vi "main.vi"() -> ()   [LabVIEW 2023]
uses:
  TypeDefs/States.ctl
  subVIs/Open_device.llb/Select_Instr.ctl
  <vilib>/Analysis/1siggen.llb/Ramp Pattern by Samples.vi
  <vilib>/Analysis/NI_AALBase.lvlib
panel:
  in  "f_start [Hz]":dbl=1.0 min=1.0 max=1000.0 format="%0.2f"
  in  "f_stop [Hz]":dbl=1.0 min=1.0 max=10000.0
  in  "samples":i32=128 min=1 max=1000
  out "Jeden punkt pomiarowy":cluster{dbl, dbl}
  out "Modul i faza impedancji":cluster{dbl, dbl}[](graph)
  out "Cosinus fi":dbl
  out "Uwagi do pomiarów":string
  out "|Z|":dbl
  out "U3 [V]":dbl format="%#.3g"
  out "U2 [V]":dbl format="%#.3g"
  out "U1 [V]":dbl format="%#.3g"
  in  "Pomiar":bool
  in  "stop":bool
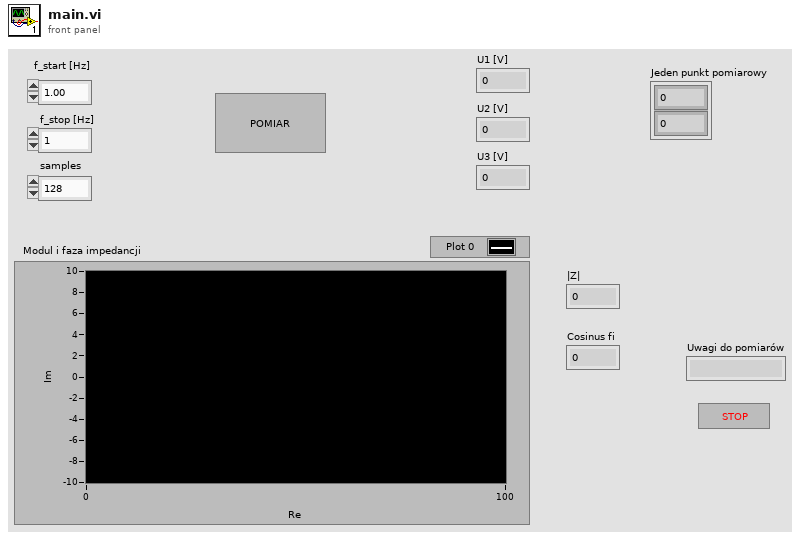
[diagram p1: front panel]
types:
  T1 = typedef "States.ctl" = enum16{"INIT", "WAIT", "EXIT", "GEN", "MEAS1", "MEAS2", "MEAS3", "CALC"}
  T2 = typedef "Select_Instr.ctl" = string
  T3 = cluster{"VISA resource name 1":refnum<visa-resource-name>, "VISA resource name 2":refnum<visa-resource-name>, "VISA resource name 3":refnum<visa-resource-name>}
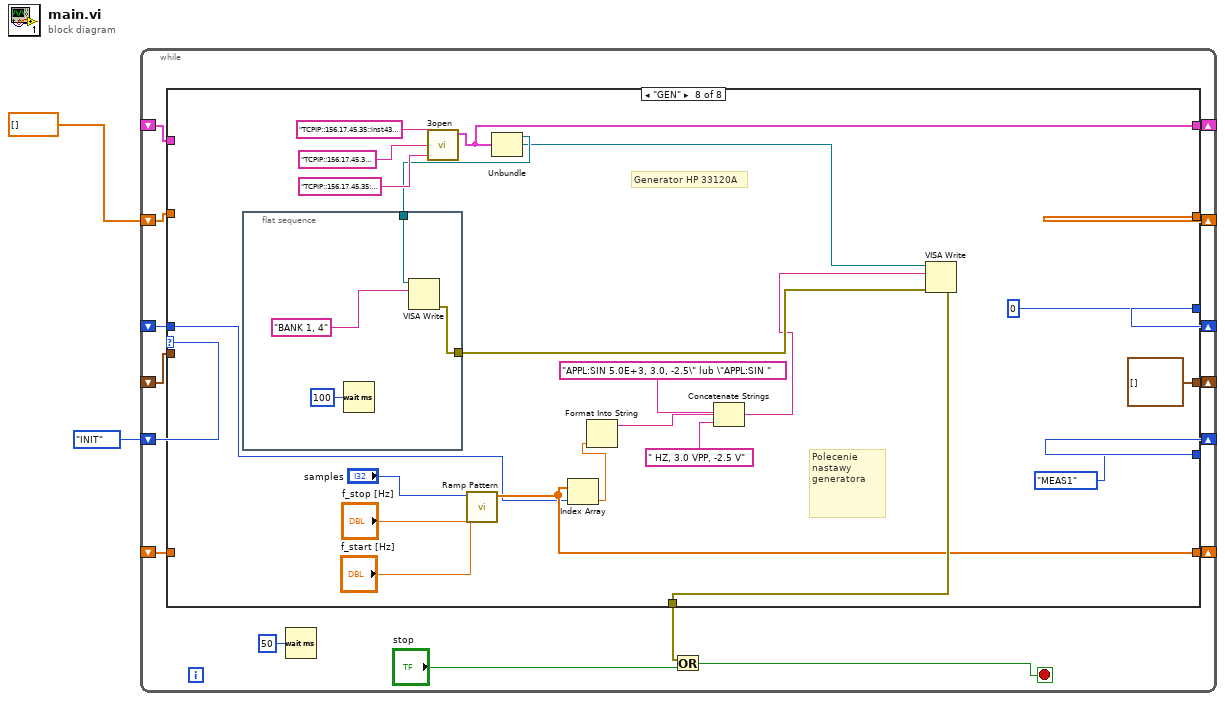
[diagram p0: block diagram]
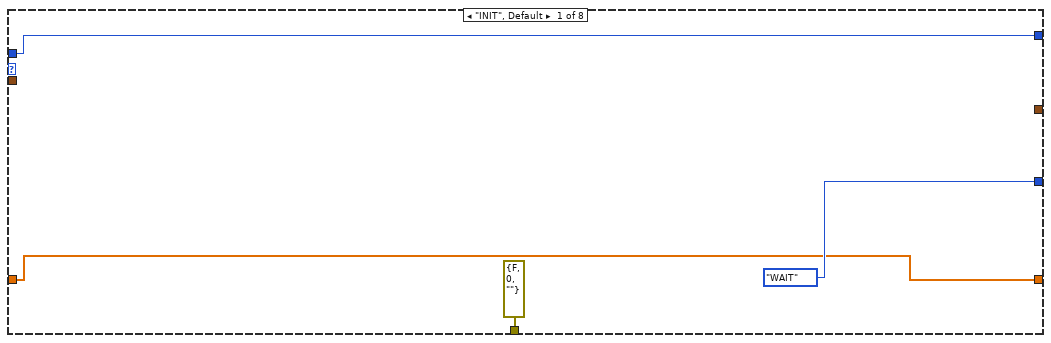
[diagram p2: hidden frame]
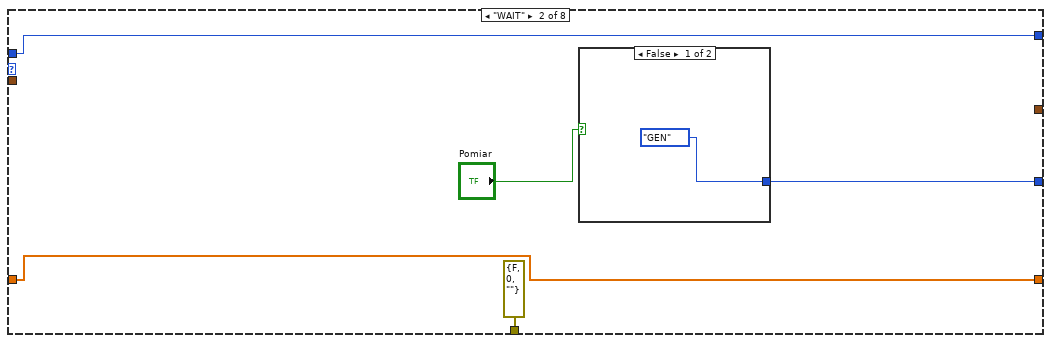
[diagram p3: hidden frame]
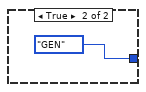
[diagram p4: hidden frame]
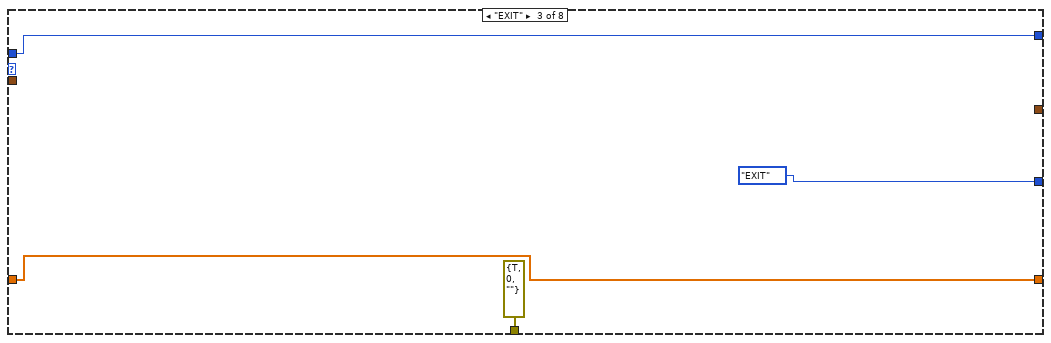
[diagram p5: hidden frame]
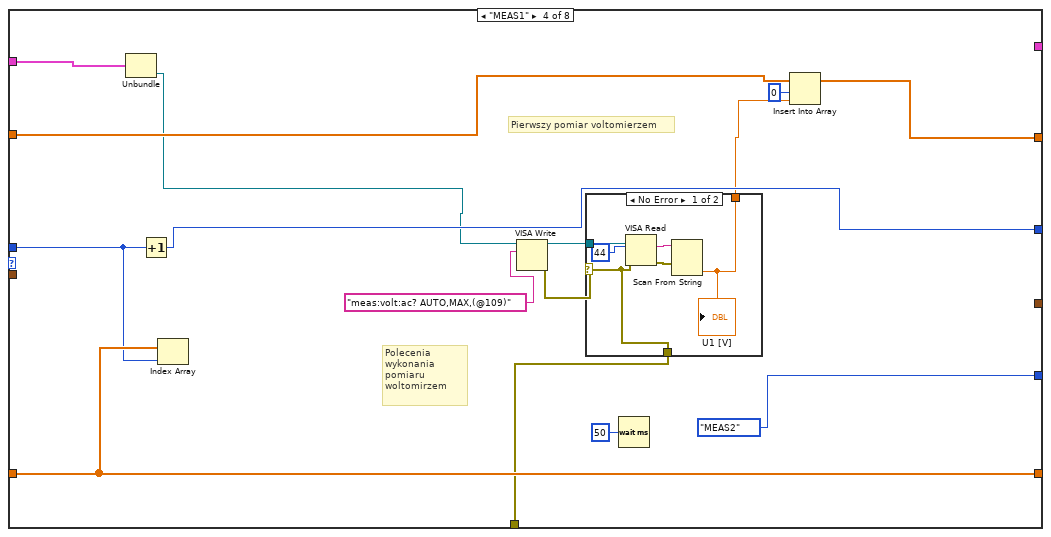
[diagram p6: hidden frame]
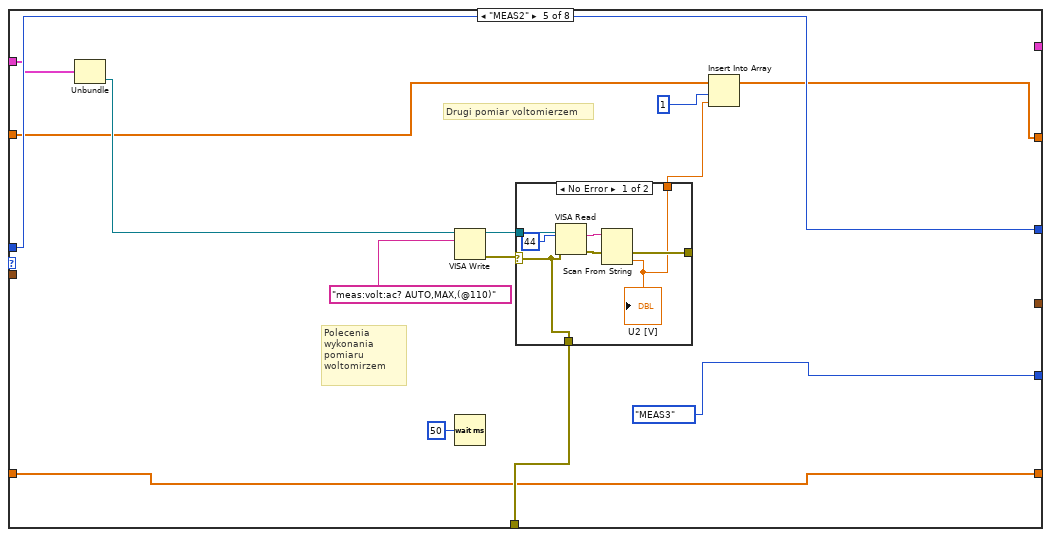
[diagram p8: hidden frame]
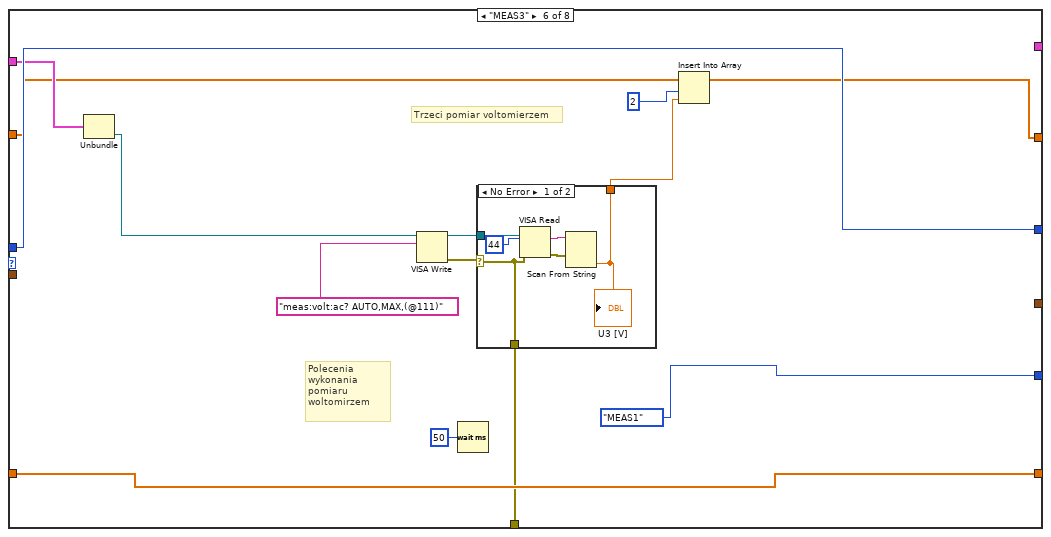
[diagram p10: hidden frame]
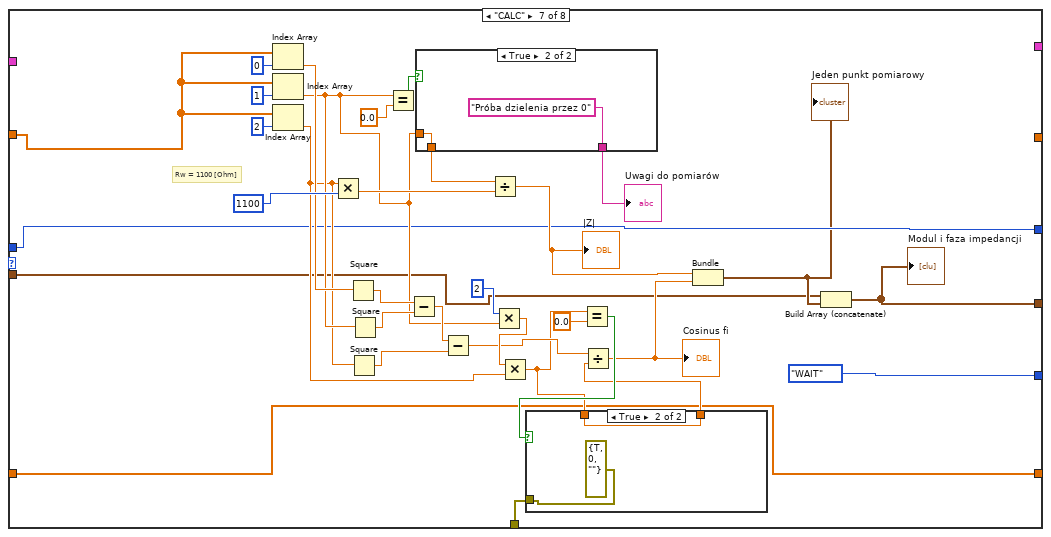
[diagram p12: hidden frame]
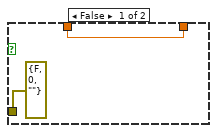
[diagram p13: hidden frame]
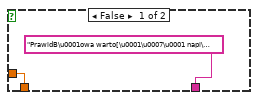
[diagram p14: hidden frame]
diagram:
  n1 = while {
    shift-right: [w18] -> _
    shift-left: States."INIT" -> [w17]
    shift-right: [w13] -> _
    shift-left: dbl[] [] -> [w12]
    shift-right: [w10] -> _
    shift-left: _ -> [w9]
    shift-right: [w8] -> _
    shift-left: _ -> [w6]
    shift-right: [w7] -> _
    shift-left: _ -> [w5]
    shift-right: [w4] -> _
    shift-left: _ -> [w3]
    stop <- w14 stop-if-true
    n2 = case shown="\"GEN\"" w17 {
      tunnel: [States."WAIT" w26 States."EXIT" States."MEAS2" States."MEAS3" States."MEAS1" States."WAIT" States."MEAS1"] -> w18
      tunnel: [errorcluster {"status"=FALSE, "code"=0, "source"=""} ("error IO") errorcluster {"status"=FALSE, "code"=0, "source"=""} ("error IO") errorcluster {"status"=TRUE, "code"=0, "source"=""} ("error IO") w35 w68 w82 w109 w148] -> w16
      tunnel: [_ _ _ w36 w56 w78 _ _] -> w13
      tunnel: w12 -> [_ _ _ w39 w59 w79 w102 _]
      tunnel: [_ _ _ _ _ _ _ w153] -> w10
      tunnel: w9 -> [_ _ _ w47 w61 w84 _ _]
      tunnel: [w20 w24 w31 w46 w67 w90 w104 w146] -> w8
      tunnel: [w19 w23 w30 w40 w66 w89 w103 0] -> w7
      tunnel: w6 -> [w20 w24 w31 w46 w67 w90 w104 _]
      tunnel: w5 -> [w19 w23 w30 w45 w66 w89 w103 w140]
      tunnel: [_ _ _ _ _ _ w99 cluster{dbl, dbl}[] []] -> w4
      tunnel: w3 -> [_ _ _ _ _ _ w100 _]
      frame "INIT", Default {
      }
      frame "WAIT" {
        n3 = case shown="False" "Pomiar" {
          tunnel: [States."GEN" States."GEN"] -> w26
          frame False {
          }
          frame True {
          }
        }
      }
      frame "EXIT" {
      }
      frame "MEAS1" {
        # "Polecenia wykonania \npomiaru woltomirzem"
        # "Pierwszy pomiar voltomierzem"
        n4 = Unbundle(w47) -> ("VISA resource name 3"=w34:refnum<visa-resource-name>)  [unwired: 2 out]
        n5 = Increment(x=w45) -> (x+1=w40:i32)
        n6 = Index Array(array=w46, index=w45) -> ()  [unwired: 1 out]
        n7 = VISA Write(VISA resource name=w34, write buffer="meas:volt:ac? AUTO,MAX,(@109)") -> (VISA resource name out=w43:refnum<visa-resource-name>, error out=w42:errorcluster)  [unwired: 1 in, 1 out]
        n8 = case shown="No Error" w42 {
          selector: w42 -> [w49 w55]
          tunnel: w43 -> [w54 _]
          tunnel: [w50 _] -> w38
          tunnel: [w49 w55] -> w35
          frame No Error {
            n9 = VISA Read(VISA resource name=w54, byte count=u32 44, error in (no error)=w49) -> (read buffer=w52:string, error out=w51:errorcluster)  [unwired: 2 out]
            n10 = Scan From String(input string=w52, error in=w51) -> (output 1=w50:dbl)  [unwired: 3 in, 3 out]
            "U1 [V]" <- w50
          }
          frame Error {
          }
        }
        n11 = Wait (ms)(milliseconds to wait=u32 50) -> ()  [unwired: 1 out]
        n12 = Insert Into Array(array=w39, index=0, new element=w38) -> (w36:dbl[])
      }
      frame "MEAS2" {
        # "Polecenia wykonania \npomiaru woltomirzem"
        # "Drugi pomiar voltomierzem"
        n13 = Unbundle(w61) -> ("VISA resource name 3"=w60:refnum<visa-resource-name>)  [unwired: 2 out]
        n14 = VISA Write(VISA resource name=w60, write buffer="meas:volt:ac? AUTO,MAX,(@110)") -> (VISA resource name out=w64:refnum<visa-resource-name>, error out=w63:errorcluster)  [unwired: 1 in, 1 out]
        n15 = Wait (ms)(milliseconds to wait=u32 50) -> ()  [unwired: 1 out]
        n16 = case shown="No Error" w63 {
          selector: w63 -> [w70 w77]
          tunnel: w64 -> [w76 _]
          tunnel: [w72 w77] -> _
          tunnel: [w71 _] -> w57
          tunnel: [w70 w77] -> w68
          frame No Error {
            n17 = VISA Read(VISA resource name=w76, byte count=u32 44, error in (no error)=w70) -> (read buffer=w74:string, error out=w73:errorcluster)  [unwired: 2 out]
            n18 = Scan From String(input string=w74, error in=w73) -> (error out=w72:errorcluster, output 1=w71:dbl)  [unwired: 3 in, 2 out]
            "U2 [V]" <- w71
          }
          frame Error {
          }
        }
        n19 = Insert Into Array(array=w59, index=1, new element=w57) -> (w56:dbl[])
      }
      frame "MEAS3" {
        # "Polecenia wykonania \npomiaru woltomirzem"
        # "Trzeci pomiar voltomierzem"
        n20 = Unbundle(w84) -> ("VISA resource name 3"=w83:refnum<visa-resource-name>)  [unwired: 2 out]
        n21 = VISA Write(VISA resource name=w83, write buffer="meas:volt:ac? AUTO,MAX,(@111)") -> (VISA resource name out=w87:refnum<visa-resource-name>, error out=w86:errorcluster)  [unwired: 1 in, 1 out]
        n22 = Wait (ms)(milliseconds to wait=u32 50) -> ()  [unwired: 1 out]
        n23 = case shown="No Error" w86 {
          selector: w86 -> [w92 w98]
          tunnel: w87 -> [w97 _]
          tunnel: [w93 _] -> w80
          tunnel: [w92 w98] -> w82
          frame No Error {
            n24 = VISA Read(VISA resource name=w97, byte count=u32 44, error in (no error)=w92) -> (read buffer=w95:string, error out=w94:errorcluster)  [unwired: 2 out]
            n25 = Scan From String(input string=w95, error in=w94) -> (output 1=w93:dbl)  [unwired: 3 in, 3 out]
            "U3 [V]" <- w93
          }
          frame Error {
          }
        }
        n26 = Insert Into Array(array=w79, index=2, new element=w80) -> (w78:dbl[])
      }
      frame "CALC" {
        # "Rw = 1100 [Ohm]"
        n27 = Index Array(array=w102, index=0) -> (element=w123:dbl)
        n28 = Index Array(array=w102, index=1) -> (element=w116:dbl)
        n29 = Index Array(array=w102, index=2) -> (element=w115:dbl)
        n30 = Multiply(x=w115, y=1100) -> (x*y=w124:dbl)
        n31 = Square(x=w123) -> (x^2=w122:dbl)
        n32 = Square(x=w115) -> (x^2=w119:dbl)
        n33 = Square(x=w116) -> (x^2=w121:dbl)
        n34 = Equal?(x=w116, y=0.0) -> (x = y?=w126:bool)
        n35 = Subtract(x=w122, y=w121) -> (x-y=w120:dbl)
        n36 = case shown="True" w126 {
          tunnel: w116 -> [w137 w139]
          tunnel: [w137 w139] -> w125
          tunnel: ["PrawidB\u0001owa warto[\u0001\u0007\u0001 napi\u0019\u0001cia" ("String") "Próba dzielenia przez 0" ("String")] -> w107
          frame False {
          }
          frame True {
          }
        }
        "Uwagi do pomiarów" <- w107
        n37 = Subtract(x=w120, y=w119) -> (x-y=w114:dbl)
        n38 = Divide(x=w125, y=w124) -> (x/y=w106:dbl)
        "|Z|" <- w106
        n39 = Multiply(x=2, y=w116) -> (x*y=w117:dbl)
        n40 = Multiply(x=w117, y=w115) -> (x*y=w111:dbl)
        n41 = Equal?(x=w111, y=0.0) -> (x = y?=w112:bool)
        n42 = case shown="True" w112 {
          tunnel: w111 -> [w132 w134]
          tunnel: [errorcluster {"status"=FALSE, "code"=0, "source"=""} ("error IO") errorcluster {"status"=TRUE, "code"=0, "source"=""} ("error IO")] -> w109
          tunnel: [w132 w134] -> w108
          frame False {
          }
          frame True {
          }
        }
        n43 = Divide(x=w114, y=w108) -> (x/y=w105:dbl)
        "Cosinus fi" <- w105
        n44 = Bundle(w106, w105) -> (w101:cluster{dbl, dbl})  [unwired: 1 in]
        "Jeden punkt pomiarowy" <- w101
        n45 = Build Array (concatenate)(w100, w101) -> (w99:cluster{dbl, dbl}[])
        "Modul i faza impedancji" <- w99
      }
      frame "GEN" {
        # "Generator HP 33120A"
        # "Polecenie nastawy generatora"
        n46 = flat-sequence {
          tunnel: [w163] -> w159
          tunnel: w155 -> [w161]
          frame #0 {
            n47 = Wait (ms)(milliseconds to wait=u32 100) -> ()  [unwired: 1 out]
            n48 = VISA Write(VISA resource name=w161, write buffer="BANK 1, 4") -> (error out=w163:errorcluster)  [unwired: 1 in, 2 out]
          }
        }
        n49 = call "3open.vi"("VISA resource name 1"=T2 "TCPIP::156.17.45.35::inst43::INSTR" ("Select_Instrument"), "VISA resource name 2"=T2 "TCPIP::156.17.45.35::inst44::INSTR" ("Select_Instrument"), "VISA resource name 3"=T2 "TCPIP::156.17.45.35::inst41::INSTR" ("Select_Instrument")) -> ("InstrCluster"=w153:T3)  [unwired: 1 in, 3 out]
        n50 = call-poly <vilib>:"Ramp Pattern.vi"("start"="f_start [Hz]", "end"="f_stop [Hz]", "samples"="samples") -> ("Ramp Pattern"=w146:dbl[])  [unwired: 7 in, 1 out]
        n51 = Unbundle(w153) -> ("VISA resource name 1"=w155:refnum<visa-resource-name>, "VISA resource name 2"=w154:refnum<visa-resource-name>)  [unwired: 1 out]
        n52 = Index Array(array=w146, index=w140) -> (element=w144:dbl)
        n53 = Format Into String(w144) -> (resulting string=w143:string)  [unwired: 3 in, 1 out]
        n54 = Concatenate Strings("APPL:SIN 5.0E+3, 3.0, -2.5\" lub \"APPL:SIN ", w143, " HZ, 3.0 VPP, -2.5 V") -> (w141:string)
        n55 = VISA Write(VISA resource name=w154, write buffer=w141, error in (no error)=w159) -> (error out=w148:errorcluster)  [unwired: 2 out]
      }
    }
    n56 = Wait (ms)(milliseconds to wait=u32 50) -> ()  [unwired: 1 out]
    n57 = Or(x=w16, y="stop") -> (x .or. y?=w14:bool)
  }
